vi "scaled_error.vi"(0 "x":dbl, 1 "x_target":dbl, 2 "y":dbl, 3 "y_target":dbl, 4 "size_m":dbl) -> (5 "err_x":dbl, 6 "err_y":dbl)   [LabVIEW 2019]
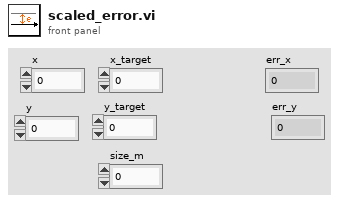
[diagram p1: front panel]
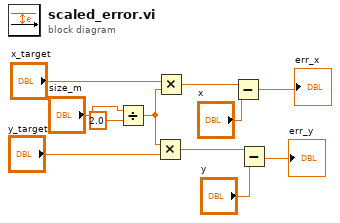
[diagram p0: block diagram]
diagram:
  n1 = Divide(x="size_m", y=2.0) -> (x/y=w9:dbl)
  n2 = Multiply(x=w9, y="y_target") -> (x*y=w4:dbl)
  n3 = Multiply(x="x_target", y=w9) -> (x*y=w6:dbl)
  n4 = Subtract(x=w6, y="x") -> (x-y=→"err_x":dbl)
  n5 = Subtract(x=w4, y="y") -> (x-y=→"err_y":dbl)
